vi "Send Load Core Sequential.vi"(5 "Class Relative Paths Path":path, 7 "Async Message Settings":T1={"Message Priority (Normal)"=enum."Normal", "Async Call Method (Call and Collect)"=enum."Call and Collect", "VI Refnum Lifetime (Destroy on Actor Exit)"=enum."Destroy on Actor Exit", "Report Errors (T)"=TRUE, "Caller Enqueuer"=refnum, "Completion Notification Msg"=refnum}, 8 "error in (no error)":errorcluster, 9 "Reference Class Path":path, 10 "Caller Enqueuer":refnum<class "Message Enqueuer.lvclass">, 11 "Message Enqueuer in":refnum<class "Message Enqueuer.lvclass">) -> (0 "error out":errorcluster, 2 "GUID":string, 3 "Message Enqueuer out":refnum<class "Message Enqueuer.lvclass">)   [LabVIEW 2023, in "Class Loader.lvlib" / "Load Core Sequential Msg.lvclass"]
doc: "Sends the <b>Class Loader.lvlib:Load Core Sequential Msg.lvclass</b> Async Message.\n\nThis message will call <b>Load Core Sequential.vi</b> on the <b>Class Loader.lvlib:Class Loader.lvclass</b> Async Method Actor.\n\n<b>Load Core Sequential.vi Description</b>"
uses:
  Load Core Sequential Msg.lvclass
  <vilib>/ActorFramework/Message Enqueuer/Message Enqueuer.lvclass
  <vilib>/LS Instruments AG/Async Methods Actor/Async Methods Actor/Async Methods Actor Messages/Async Message/Async Message Settings.ctl
  <vilib>/LS Instruments AG/Async Methods Actor/Async Methods Actor/Async Methods Actor Messages/Completion Notification Msg/Completion Notification Msg.lvclass
  <vilib>/ActorFramework/Message Enqueuer/Message Priority.ctl
  <vilib>/LS Instruments AG/Async Methods Actor/Async Methods Actor/Async Methods Actor/Async Call Method.ctl
  <vilib>/LS Instruments AG/Async Methods Actor/Async Methods Actor/Async Methods Actor/VI Refnum Lifetime.ctl
  C:/Program Files/National Instruments/LabVIEW 2025/vi.lib/LS Instruments AG/Async Methods Actor/Async Methods Actor/Async Methods Actor Messages/Async Message/Async Message.lvclass
  Load Core Sequential Msg.lvclass/Load Core Sequential Msg.ctl
  <vilib>/LS Instruments AG/Async Methods Actor/Async Methods Actor/Async Methods Actor Messages/Async Message/Async Message.lvclass/Async Message.ctl
  <vilib>/ActorFramework/Message Enqueuer/Message Enqueuer.lvclass/Message Enqueuer.ctl
  <vilib>/LS Instruments AG/Async Methods Actor/Async Methods Actor/Async Methods Actor Messages/Async Message/Write Caller Enqueuer.vi
  <vilib>/LS Instruments AG/Async Methods Actor/Async Methods Actor/Async Methods Actor Messages/Async Message/Write Completion Notification Msg.vi
  <vilib>/ActorFramework/Message Enqueuer/Enqueue.vi
  <vilib>/LS Instruments AG/Async Methods Actor/Async Methods Actor/Async Methods Actor Messages/Async Message/Async Message.lvclass
  C:/Program Files/National Instruments/LabVIEW 2025/vi.lib/ActorFramework/Message/Message.lvclass
  <vilib>/string/Create NI GUID.vi
  <vilib>/ActorFramework/Message Priority Queue/Priority Enqueue.vi
  <vilib>/LS Instruments AG/Async Methods Actor/Async Methods Actor/Async Methods Actor/Async Methods Actor.lvclass
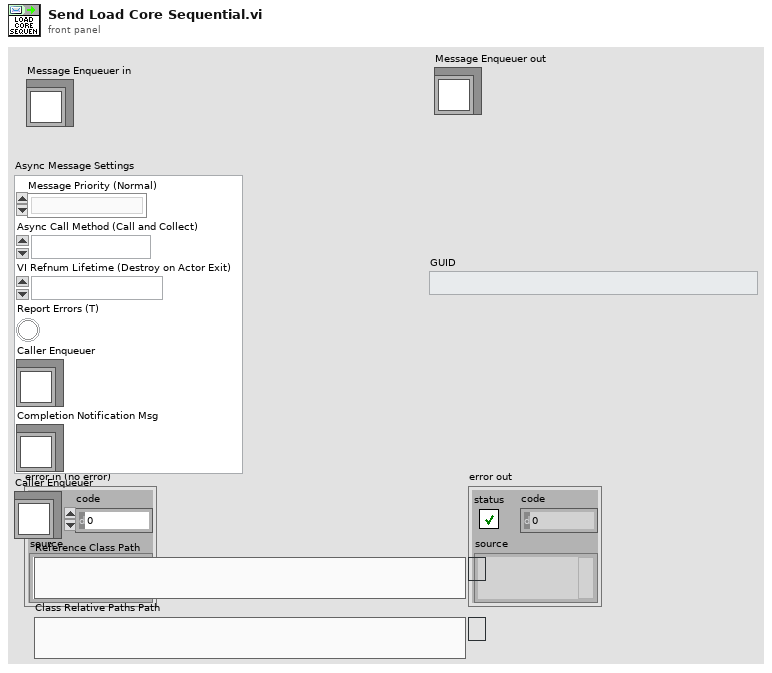
[diagram p1: front panel]
types:
  T1 = typedef "Async Methods Actor.lvlib/Async Message.lvclass/Async Message Settings.ctl" = cluster{"Message Priority (Normal)":T2, "Async Call Method (Call and Collect)":T3, "VI Refnum Lifetime (Destroy on Actor Exit)":T4, "Report Errors (T)":bool, "Caller Enqueuer":refnum<class "Message Enqueuer.lvclass">, "Completion Notification Msg":refnum<class "Completion Notification Msg.lvclass">}
  T2 = typedef "Actor Framework.lvlib/Message Enqueuer.lvclass/Message Priority.ctl" = enum16{"Low", "Normal", "High"}
  T3 = typedef "Async Methods Actor.lvlib/Async Methods Actor.lvclass/Async Call Method.ctl" = enum16{"Call and Collect", "Call and Forget"}
  T4 = typedef "Async Methods Actor.lvlib/Async Methods Actor.lvclass/VI Refnum Lifetime.ctl" = enum16{"Destroy on Exit", "Destroy on Actor Exit", "Destroy on Application Exit"}
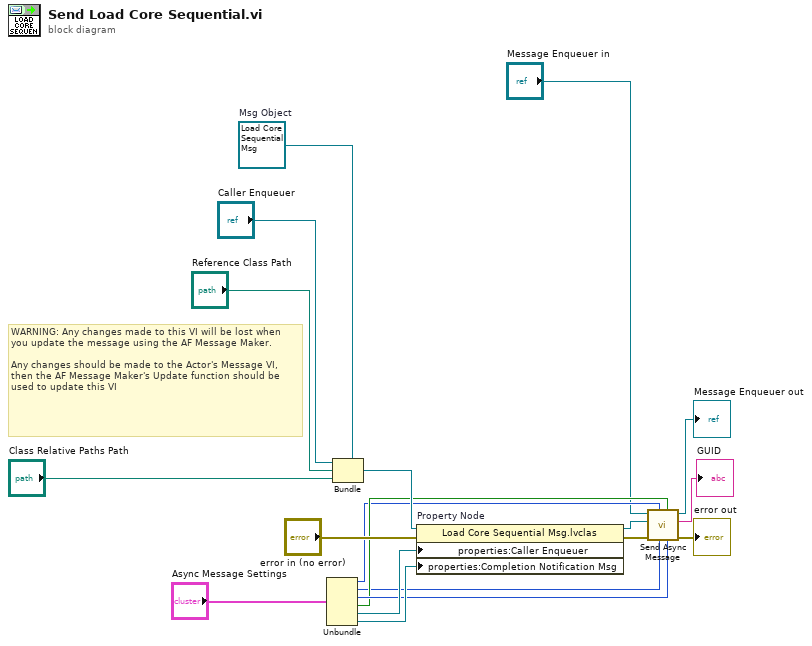
[diagram p0: block diagram]
diagram:
  w15 = refnum<class "Load Core Sequential Msg.lvclass"> refnum  # Msg Object
  # "WARNING: Any changes made to this VI will be lost when you update the message using the AF Message Maker.\n\nAny changes should be made to the Actor's Message VI, then the AF Message Maker's Update function should be used to update this VI"
  n1 = Unbundle "Unbundle"("Async Message Settings") -> ("Message Priority (Normal)"=w4:T2, "Async Call Method (Call and Collect)"=w5:T3, "VI Refnum Lifetime (Destroy on Actor Exit)"=w7:T4, "Report Errors (T)"=w6:bool, "Caller Enqueuer"=w12:refnum<class "Message Enqueuer.lvclass">, "Completion Notification Msg"=w11:refnum<class "Completion Notification Msg.lvclass">)
  n2 = Bundle(cluster=w15, "Caller Enqueuer", "Reference Class Path", "Class Relative Paths Path") -> (w13:refnum<class "Load Core Sequential Msg.lvclass">)
  n3 = property on="Property Node" class="Load Core Sequential Msg.lvclas"(reference=w13, error in="error in (no error)", "properties:Caller Enqueuer"=w12, "properties:Completion Notification Msg"=w11) -> (reference out=w2:refnum<class "Load Core Sequential Msg.lvclass">, error out=w3:errorcluster)
  n4 = call <vilib>:"Send Async Message.vi"("VI Refnum Lifetime (Destroy on Actor Exit)"=w7, "Report Errors (T)"=w6, "Async Call Method (Call and Collect)"=w5, "Message Priority (Normal)"=w4, "error in (no error)"=w3, "Concrete Async Message"=w2, "Message Enqueuer"="Message Enqueuer in") -> ("error out"=→"error out":errorcluster, "GUID"=→"GUID":string, "Message Enqueuer out"=→"Message Enqueuer out":refnum<class "Message Enqueuer.lvclass">)  [unwired: 2 in]
